vi "DMM 3446X Measure Multiple.vi"(4 "Absolute Resolution":dbl=1e-06, 6 "Timeout (10000 ms)":i32=10000 format="%#.6g", 8 "error in (no error)":errorcluster, 9 "Sample Count (1)":i32=1, 10 "Measurement Function (10: Voltage DC)":i32(ring)=10 items=["Continuity", "Current AC", "Current DC", "Diode", "Frequency", "Resistance 4-wire", "Period", "Resistance 2-wire", "Temperature", "Voltage AC", "Voltage DC", "Voltage DC Ratio"], 11 "VISA resource name":refnum<visa-resource-name>) -> (0 "error out":errorcluster, 3 "Measurements":dbl[](array[numeric]))   [LabVIEW 2018]
doc: "This example shows how to configure a measurement and take multiple readings."
uses:
  <instrlib>/Agilent 3446X Series/Public/Data/Read (Multiple Points).vi
  <instrlib>/Agilent 3446X Series/Agilent 3446X Series.lvlib
panel:
  in  "Manual Range (1)":dbl=1.0
  in  "Auto Range":bool=TRUE
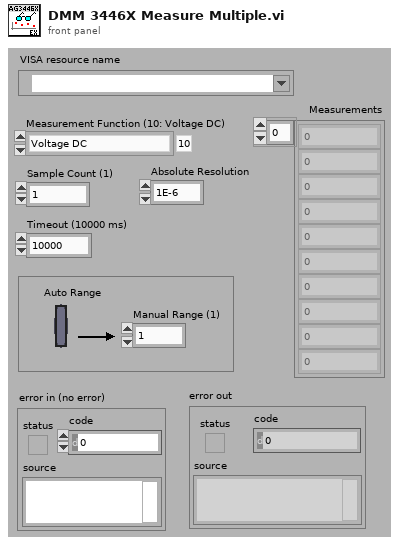
[diagram p1: front panel]
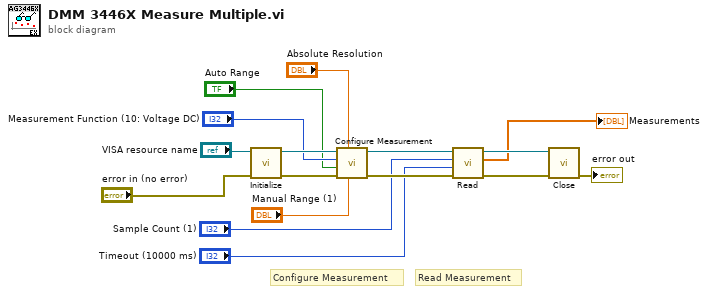
[diagram p0: block diagram]
diagram:
  # "Read Measurement"
  # "Configure Measurement"
  n1 = call <instrlib>:"Initialize.vi"("error in (no error)"="error in (no error)", "VISA resource name"="VISA resource name") -> ("error out"=w15:errorcluster, "VISA resource name out"=w16:refnum<visa-resource-name>)  [unwired: 3 in, 5 out]
  n2 = call <instrlib>:"Configure Measurement.vi"("Manual Range (1)"="Manual Range (1)", "Absolute Resolution (1E-6)"="Absolute Resolution", "error in (no error)"=w15, "Auto Range (T: Enable)"="Auto Range", "Measurement Function (10: Voltage DC)"="Measurement Function (10: Voltage DC)", "VISA resource name"=w16) -> ("error out"=w13:errorcluster, "VISA resource name out"=w12:refnum<visa-resource-name>)  [unwired: 4 out]
  n3 = call-poly <instrlib>:"Read.vi"("error in (no error)"=w13, "Timeout (10000 ms)"="Timeout (10000 ms)", "Sample Count (1)"="Sample Count (1)", "VISA resource name"=w12) -> ("error out"=w14:errorcluster, "Measurements"=→"Measurements":dbl[], "VISA resource name out"=w11:refnum<visa-resource-name>)  [unwired: 5 out]
  n4 = call <instrlib>:"Close.vi"("error in (no error)"=w14, "VISA resource name"=w11) -> ("error out"=→"error out":errorcluster)  [unwired: 9 out]
